vi "FTW-ZMQ-LibraryReturnValue.vi"(0 "error in":errorcluster, 2 "Error Message":string, 7 "Return Value":i32) -> (4 "error out":errorcluster)   [LabVIEW 2012, in "FTW-Actor.lvlib" / "FTW-Endpoint-ZMQ.lvclass"]
uses:
  FTW-Endpoint-ZMQ.lvclass
panel:
  # "Inputs"
  # "Outputs"
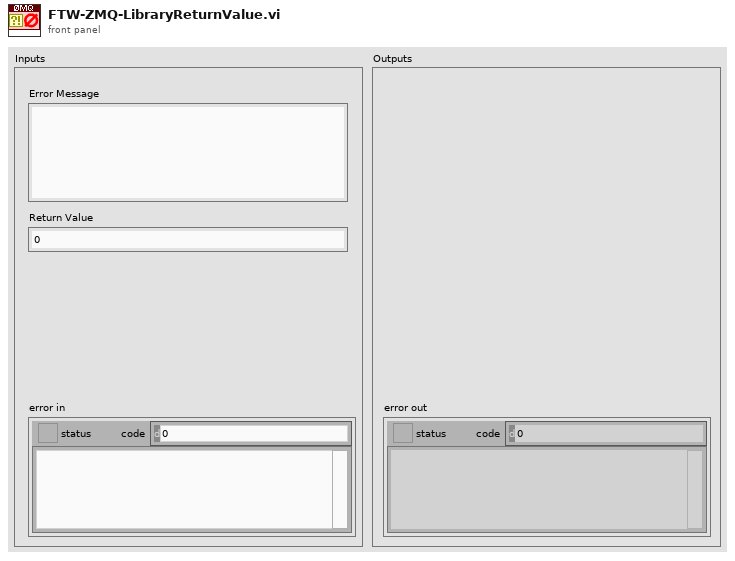
[diagram p1: front panel]
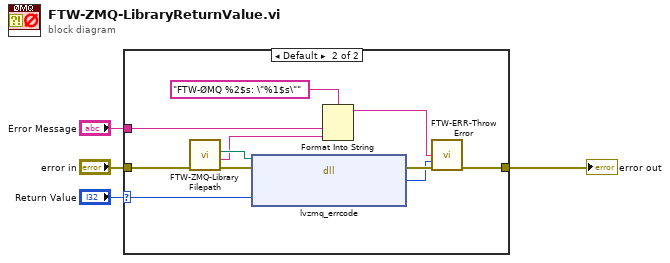
[diagram p0: block diagram]
diagram:
  n1 = case shown="Default" "Return Value" {
    selector: "Return Value" -> [_ w10]
    tunnel: "error in" -> [w5 w16]
    tunnel: [w5 w14] -> w3
    tunnel: "Error Message" -> [_ w6]
    frame 0 {
    }
    frame Default {
      n2 = call "FTW-ZMQ-LibraryFilepath.vi"("error in"=w16) -> ("error out"=w9:errorcluster, "ØMQ Version"=w7:string, "FTW-ZMQ Library Filepath"=w8:path)  [unwired: 8 in]
      n3 = dll-call lib="?" fn="lvzmq_errcode" ("zmq_labview.dll:lvzmq_strerror")(path in=w8, error in=w9, "Error Code from FTW-ZMQ"=w10) -> (error out=w15:errorcluster, "LabVIEW Error Code"=w13:i32)  [unwired: 2 in, 1 out]
      n4 = Format Into String(format string="FTW-ØMQ %2$s: \"%1$s\"" ("Error Message"), w6, w7) -> (resulting string=w11:string)  [unwired: 2 in, 1 out]
      n5 = call "FTW-ERR-ThrowError.vi"("Error Message"=w11, "Error Code"=w13, "error in"=w15) -> ("error out"=w14:errorcluster)  [unwired: 12 in]
    }
  }
  "error out" <- w3
